vi "sensor integration for debug v4.vi"() -> ()   [LabVIEW 2021]
uses:
  controls/sensirion_flow_sensor_data.ctl
  65c7c016-c5e7-4ca0-8b30-908e1d77d521.vi
  <vilib>/Analysis/baseanly.llb/Mean (DBL).vi
  <vilib>/Instr/_visa.llb/VISA Configure Serial Port (Instr).vi
  <vilib>/Analysis/NI_AALBase.lvlib
panel:
  out "logfile size (in MB)":dbl format="%.2f"
  out "sensirion data string":string
  in  "error in (no error)":errorcluster
  out "retry count":i32
  in  "read byte count (512)":u32=512
  in  "baud rate (576000)":u32=576000
  out "last loop time, ms":dbl
  out "mean refresh rate, Hz, n=50":dbl
  in  "loop delay, ms (0)":u32
  in  "expected num sensors (12)":i32=12
  out "sensor data array 7 - 12":T1[](array[typedef])=[{"flow rate \n(mL/min)"=0.0, "flow val. status"=FALSE, "temp.\n(C)"=0.0, "temp. val status"=FALSE, "air in \nline?"=FALSE, "high \nflow?"=FALSE, "flag. val status"=FALSE}, {"flow rate \n(mL/min)"=0.0, "flow val. status"=FALSE, "temp.\n(C)"=0.0, "temp. val status"=FALSE, "air in \nline?"=FALSE, "high \nflow?"=FALSE, "flag. val status"=FALSE}, {"flow rate \n(mL/min)"=0.0, "flow val. status"=TRUE, "temp.\n(C)"=0.0, "temp. val status"=TRUE, "air in \nline?"=FALSE, "high \nflow?"=FALSE, "flag. val status"=TRUE}, {"flow rate \n(mL/min)"=0.0, "flow val. status"=TRUE, "temp.\n(C)"=0.0, "temp. val status"=TRUE, "air in \nline?"=FALSE, "high \nflow?"=FALSE, "flag. val status"=TRUE}, {"flow rate \n(mL/min)"=0.0, "flow val. status"=TRUE, "temp.\n(C)"=0.0, "temp. val status"=TRUE, "air in \nline?"=FALSE, "high \nflow?"=FALSE, "flag. val status"=TRUE}, {"flow rate \n(mL/min)"=0.0, "flow val. status"=TRUE, "temp.\n(C)"=0.0, "temp. val status"=TRUE, "air in \nline?"=FALSE, "high \nflow?"=FALSE, "flag. val status"=TRUE}, {"flow rate \n(mL/min)"=0.0, "flow val. status"=TRUE, "temp.\n(C)"=0.0, "temp. val status"=TRUE, "air in \nline?"=FALSE, "high \nflow?"=FALSE, "flag. val status"=TRUE}, {"flow rate \n(mL/min)"=0.0, "flow val. status"=TRUE, "temp.\n(C)"=0.0, "temp. val status"=TRUE, "air in \nline?"=FALSE, "high \nflow?"=FALSE, "flag. val status"=TRUE}, {"flow rate \n(mL/min)"=0.0, "flow val. status"=TRUE, "temp.\n(C)"=0.0, "temp. val status"=TRUE, "air in \nline?"=FALSE, "high \nflow?"=FALSE, "flag. val status"=TRUE}, {"flow rate \n(mL/min)"=0.0, "flow val. status"=TRUE, "temp.\n(C)"=0.0, "temp. val status"=TRUE, "air in \nline?"=FALSE, "high \nflow?"=FALSE, "flag. val status"=TRUE}, {"flow rate \n(mL/min)"=0.0, "flow val. status"=TRUE, "temp.\n(C)"=0.0, "temp. val status"=TRUE, "air in \nline?"=FALSE, "high \nflow?"=FALSE, "flag. val status"=TRUE}, {"flow rate \n(mL/min)"=0.0, "flow val. status"=TRUE, "temp.\n(C)"=0.0, "temp. val status"=TRUE, "air in \nline?"=FALSE, "high \nflow?"=FALSE, "flag. val status"=TRUE}] {"temp.\n(C)" scale=20.0..30.0 scale format="%#_3g"; "flow rate \n(mL/min)" scale=0.0..4.0}
  out "sensor data array 1 - 6":T1[](array[typedef])=[{"flow rate \n(mL/min)"=0.0, "flow val. status"=FALSE, "temp.\n(C)"=0.0, "temp. val status"=FALSE, "air in \nline?"=FALSE, "high \nflow?"=FALSE, "flag. val status"=FALSE}, {"flow rate \n(mL/min)"=0.0, "flow val. status"=FALSE, "temp.\n(C)"=0.0, "temp. val status"=FALSE, "air in \nline?"=FALSE, "high \nflow?"=FALSE, "flag. val status"=FALSE}, {"flow rate \n(mL/min)"=0.0, "flow val. status"=TRUE, "temp.\n(C)"=0.0, "temp. val status"=TRUE, "air in \nline?"=FALSE, "high \nflow?"=FALSE, "flag. val status"=TRUE}, {"flow rate \n(mL/min)"=0.0, "flow val. status"=TRUE, "temp.\n(C)"=0.0, "temp. val status"=TRUE, "air in \nline?"=FALSE, "high \nflow?"=FALSE, "flag. val status"=TRUE}, {"flow rate \n(mL/min)"=0.0, "flow val. status"=TRUE, "temp.\n(C)"=0.0, "temp. val status"=TRUE, "air in \nline?"=FALSE, "high \nflow?"=FALSE, "flag. val status"=TRUE}, {"flow rate \n(mL/min)"=0.0, "flow val. status"=TRUE, "temp.\n(C)"=0.0, "temp. val status"=TRUE, "air in \nline?"=FALSE, "high \nflow?"=FALSE, "flag. val status"=TRUE}, {"flow rate \n(mL/min)"=0.0, "flow val. status"=TRUE, "temp.\n(C)"=0.0, "temp. val status"=TRUE, "air in \nline?"=FALSE, "high \nflow?"=FALSE, "flag. val status"=TRUE}, {"flow rate \n(mL/min)"=0.0, "flow val. status"=TRUE, "temp.\n(C)"=0.0, "temp. val status"=TRUE, "air in \nline?"=FALSE, "high \nflow?"=FALSE, "flag. val status"=TRUE}, {"flow rate \n(mL/min)"=0.0, "flow val. status"=TRUE, "temp.\n(C)"=0.0, "temp. val status"=TRUE, "air in \nline?"=FALSE, "high \nflow?"=FALSE, "flag. val status"=TRUE}, {"flow rate \n(mL/min)"=0.0, "flow val. status"=TRUE, "temp.\n(C)"=0.0, "temp. val status"=TRUE, "air in \nline?"=FALSE, "high \nflow?"=FALSE, "flag. val status"=TRUE}, {"flow rate \n(mL/min)"=0.0, "flow val. status"=TRUE, "temp.\n(C)"=0.0, "temp. val status"=TRUE, "air in \nline?"=FALSE, "high \nflow?"=FALSE, "flag. val status"=TRUE}, {"flow rate \n(mL/min)"=0.0, "flow val. status"=TRUE, "temp.\n(C)"=0.0, "temp. val status"=TRUE, "air in \nline?"=FALSE, "high \nflow?"=FALSE, "flag. val status"=TRUE}] {"temp.\n(C)" scale=20.0..30.0 scale format="%#_3g"; "flow rate \n(mL/min)" scale=0.0..3.0}
  out "error out":errorcluster
  in  "stop program":bool
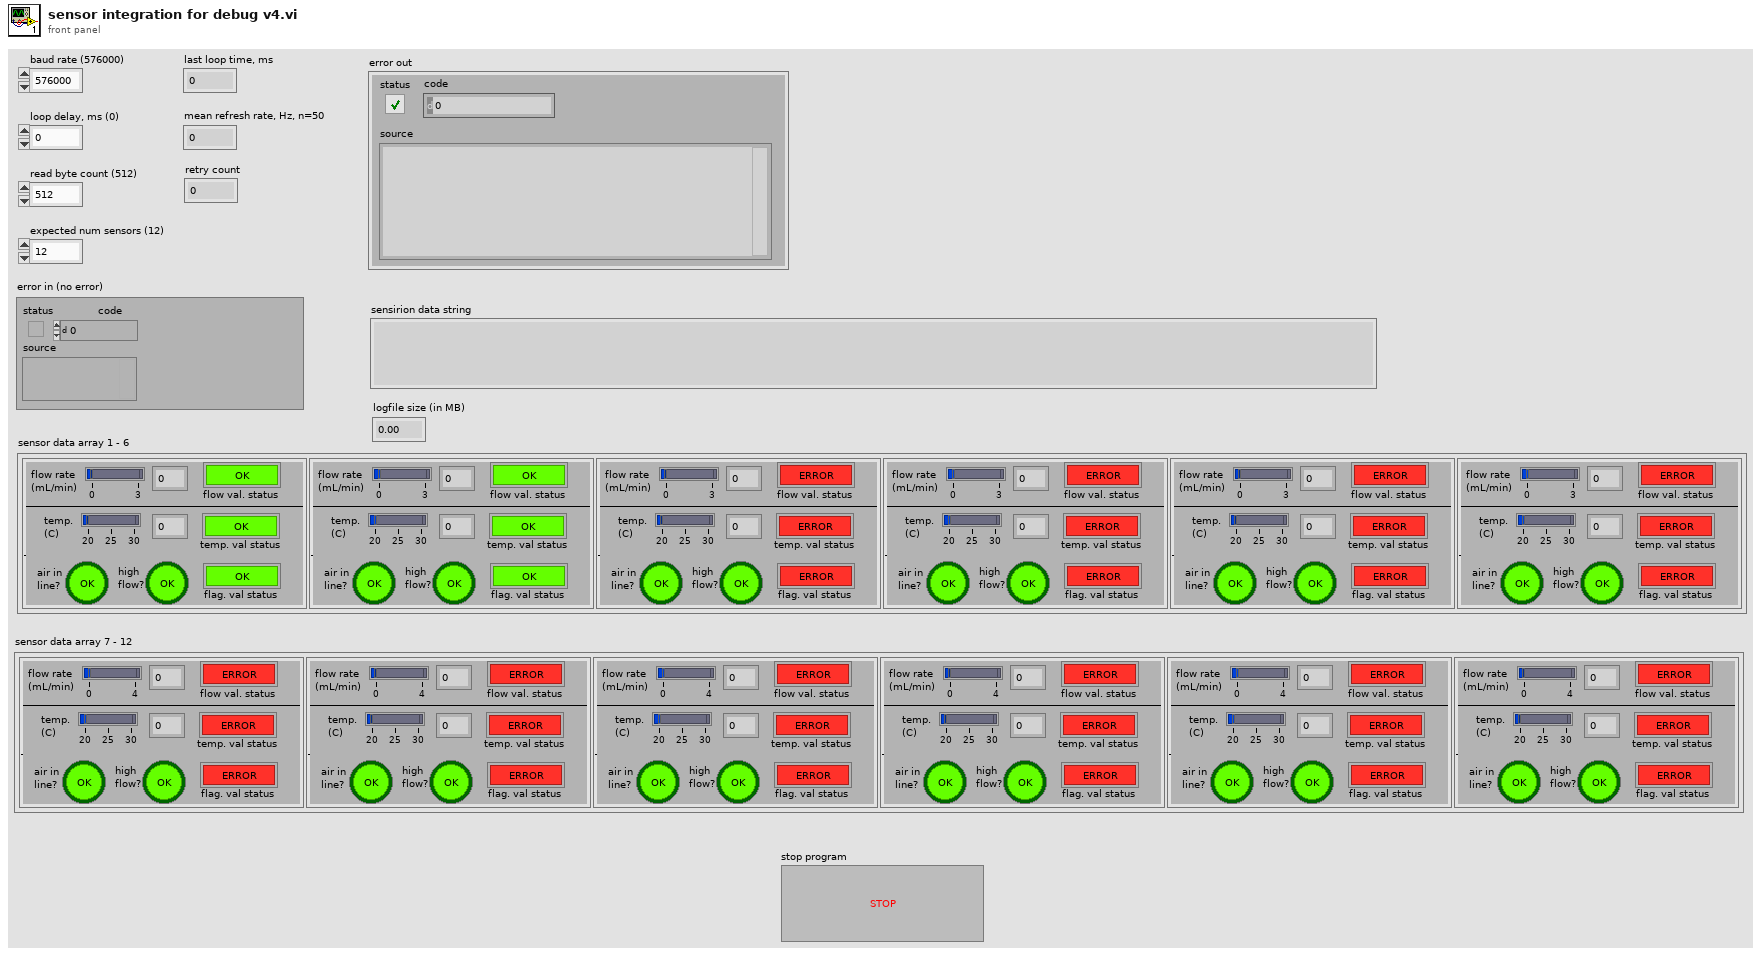
[diagram p1: front panel]
types:
  T1 = typedef "sensirion_flow_sensor_data.ctl" = cluster{"flow rate \n(mL/min)":dbl, "flow val. status":bool, "temp.\n(C)":dbl, "temp. val status":bool, "air in \nline?":bool, "high \nflow?":bool, "flag. val status":bool}
  T2 = enum16{"open", "replace", "create", "open or create", "replace or create", "replace or create with confirmation"}
  T3 = enum8{"Enabled", "Disabled", "Disabled and Grayed Out"}
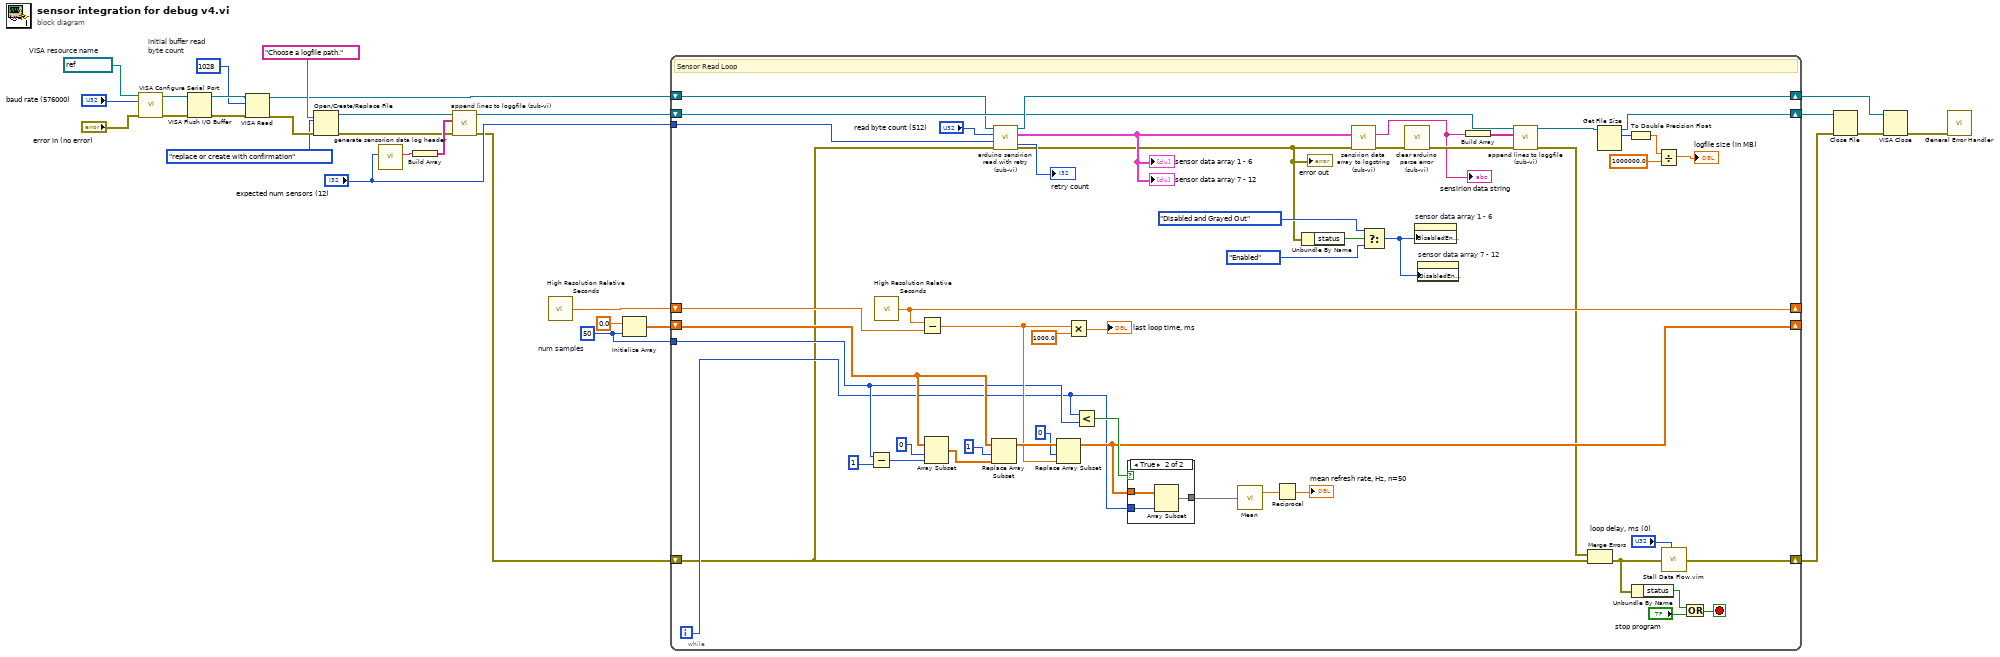
[diagram p0: block diagram]
diagram:
  w18 = 50  # num samples
  w21 = u32 1028  # initial buffer read byte count
  w26 = refnum<visa-resource-name> "COM3"  # VISA resource name
  n1 = call-poly "VISA Configure Serial Port"("VISA resource name"=w26, "baud rate (9600)"="baud rate (576000)", "error in (no error)"="error in (no error)") -> ("VISA resource name out"=w25:refnum<visa-resource-name>, "error out"=w24:errorcluster)  [unwired: 11 in]
  n2 = VISA Flush I/O Buffer(VISA resource name=w25, error in (no error)=w24) -> (VISA resource name out=w22:refnum<visa-resource-name>, error out=w23:errorcluster)  [unwired: 1 in]
  n3 = VISA Read(VISA resource name=w22, byte count=w21, error in (no error)=w23) -> (VISA resource name out=w2:refnum<visa-resource-name>, error out=w14:errorcluster)  [unwired: 2 out]
  n4 = Open/Create/Replace File(error in=w14, prompt="Choose a logfile path.", operation (0:open)=T2."replace or create with confirmation") -> (refnum out=w6:refnum<file>, error out=w4:errorcluster)  [unwired: 3 in, 1 out]
  n5 = call "generate sensorion data log header.vi"("num sensors"="expected num sensors (12)") -> ("sensor data header string"=w8:string)  [unwired: 10 in]
  n6 = Build Array(w8) -> (w7:string[])
  n7 = call "append lines to loggfile (sub-vi).vi"("error in (no error)"=w4, "string array"=w7, "file refnum"=w6) -> ("error out"=w3:errorcluster, "file refnum out"=w5:refnum<file>)  [unwired: 7 in]
  n8 = call <vilib>:"High Resolution Relative Seconds.vi"() -> ("relative seconds"=w17:dbl)
  n9 = Initialize Array(0.0 ("element"), w18) -> (w19:dbl[])
  n10 = while {
    shift-right: [w77] -> _
    shift-left: w17 -> [w76]
    shift-right: [w64] -> _
    shift-left: w19 -> [w72]
    shift-right: [w51] -> w11
    shift-left: w3 -> [w48]
    tunnel: w18 -> [w66]
    shift-right: [w33] -> w12
    shift-left: w5 -> [w36]
    tunnel: "expected num sensors (12)" -> [w37]
    shift-right: [w47] -> w28
    shift-left: w2 -> [w35]
    i -> [w63]
    stop <- w57 stop-if-true
    # "Sensor Read Loop"
    n11 = Subtract(x=w66, y=1) -> (x-y=w70:i32)
    n12 = call <vilib>:"High Resolution Relative Seconds.vi"() -> ("relative seconds"=w77:dbl)
    n13 = Subtract(x=w77, y=w76) -> (x-y=w68:dbl)
    n14 = Array Subset(array=w72, index=0, length=w70) -> (w75:dbl[])
    n15 = Replace Array Subset(array=w72, new element=w75, index=1) -> (w69:dbl[])
    n16 = call "arduino sensirion read with retry (sub-vi).vi"("error in (no error)"=w48, "expected num sensors (12)"=w37, "read byte count (512)"="read byte count (512)", "VISA resource name"=w35) -> ("error out"=w43:errorcluster, "sensor data array"=w45:T1[], "VISA resource name out"=w47:refnum<visa-resource-name>, "retry count"=→"retry count":i32)  [unwired: 4 in]
    "error out" <- w43
    "sensor data array 1 - 6" <- w45
    "sensor data array 7 - 12" <- w45
    n17 = Replace Array Subset(array=w69, new element=w68, index=0) -> (w64:dbl[])
    n18 = Multiply(x=w68, y=1000.0) -> (x*y=→"last loop time, ms":dbl)
    n19 = Less?(x=w63, y=w66) -> (x < y?=w65:bool)
    n20 = case shown="True" w65 {
      tunnel: w64 -> [w79 w82]
      tunnel: w63 -> [_ w81]
      tunnel: [w79 w80] -> w62
      frame False {
      }
      frame True {
        n21 = Array Subset(array=w82, length=w81) -> (w80:dbl[])  [unwired: 1 in]
      }
    }
    n22 = call-poly <vilib>:"Mean.vi"("X"=w62) -> ("mean"=w61:dbl)  [unwired: 1 out]
    n23 = Reciprocal(x=w61) -> (1/x=→"mean refresh rate, Hz, n=50":dbl)
    n24 = Unbundle By Name(w43) -> ("status"=w60:bool)
    n25 = call "sensirion data array to logstring (sub-vi).vi"("error in"=w43, "sensor data array"=w45) -> ("error out"=w42:errorcluster, "string out"=w38:string)  [unwired: 8 in]
    "sensirion data string" <- w38
    n26 = Select(t=T3."Disabled and Grayed Out" ("Disabled"), s=w60, f=T3."Enabled" ("Disabled")) -> (s? t:f=w58:T3)
    n27 = call "clear arduino parse error (sub-vi).vi"("error in"=w42) -> ("error out"=w41:errorcluster)  [unwired: 10 in]
    n28 = property on="sensor data array 1 - 6" class="Arr (strict)"("DisabledEnum"=w58) -> ()  [unwired: 2 in, 2 out]
    n29 = property on="sensor data array 7 - 12" class="Arr (strict)"("DisabledEnum"=w58) -> ()  [unwired: 2 in, 2 out]
    n30 = Build Array(w38) -> (w39:string[])
    n31 = call "append lines to loggfile (sub-vi).vi"("error in (no error)"=w41, "string array"=w39, "file refnum"=w36) -> ("error out"=w40:errorcluster, "file refnum out"=w34:refnum<file>)  [unwired: 7 in]
    n32 = Merge Errors(w40, w48) -> (w44:errorcluster)
    n33 = Get File Size(file=w34) -> (refnum out=w33:refnum<file>, size (in bytes)=w32:i64)  [unwired: 1 in, 1 out]
    n34 = To Double Precision Float(number=w32) -> (double precision float=w31:dbl)
    n35 = Unbundle By Name(w44) -> ("status"=w55:bool)
    n36 = Divide(x=w31, y=1000000.0) -> (x/y=→"logfile size (in MB)":dbl)
    n37 = call "Stall Data Flow.vim"("value in"=w44, "milliseconds to wait"="loop delay, ms (0)") -> ("value out"=w51:errorcluster)  [unwired: 1 out]
    n38 = Or(x=w55, y="stop program") -> (x .or. y?=w57:bool)
  }
  n39 = Close File(refnum=w12, error in=w11) -> (error out=w10:errorcluster)  [unwired: 1 out]
  n40 = VISA Close(VISA resource name=w28, error in (no error)=w10) -> (error out=w16:errorcluster)
  n41 = call <vilib>:"General Error Handler.vi"("error in (no error)"=w16) -> ()  [unwired: 10 in, 5 out]
